vi "move_andor_files.vi"(8 "error in":errorcluster, 10 "Data Files Path":path, 11 "Andor setup":T1) -> (0 "error out":errorcluster)   [LabVIEW 2012]
uses:
  Andor_settings.ctl
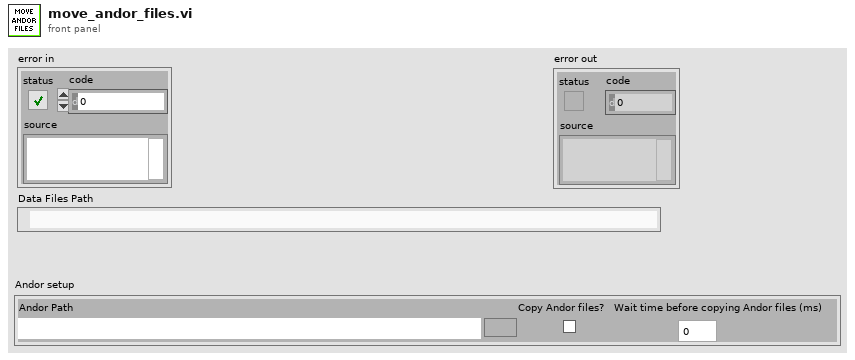
[diagram p1: front panel]
types:
  T1 = typedef "Andor_settings.ctl" = cluster{"Andor Path":path, "Copy any Andor files":bool, "Wait time before copying Andor files (ms)":u16}
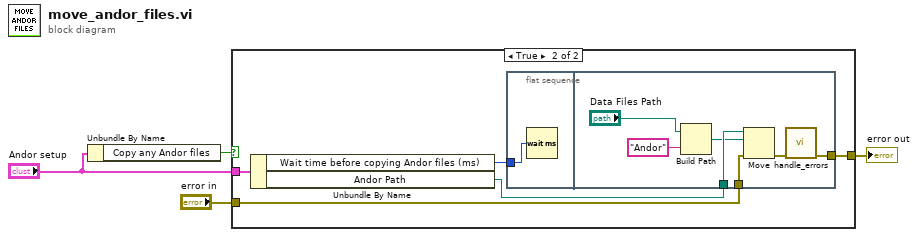
[diagram p0: block diagram]
diagram:
  n1 = Unbundle By Name("Andor setup") -> ("Copy any Andor files"=w4:bool)
  n2 = case shown="True" w4 {
    tunnel: "Andor setup" -> [_ w10]
    tunnel: "error in" -> [w5 w7]
    tunnel: [w5 w6] -> w1
    frame False {
    }
    frame True {
      n3 = Unbundle By Name(w10) -> ("Wait time before copying Andor files (ms)"=w9:u16, "Andor Path"=w8:path)
      n4 = flat-sequence {
        tunnel: w9 -> [w11]
        tunnel: w8 -> [w18]
        tunnel: w7 -> [w16]
        tunnel: [w15] -> w6
        frame #0 {
          n5 = Wait (ms)(milliseconds to wait=w11) -> ()  [unwired: 1 out]
        }
        frame #1 {
          n6 = Build Path(base path="Data Files Path", name or relative path="Andor") -> (appended path=w12:path)
          n7 = Move(source path=w18, error in=w16, 10:w12) -> (error out=w17:errorcluster)  [unwired: 2 in, 2 out]
          n8 = call "handle_errors.vi"("error in (no error)"=w17) -> ("error out"=w15:errorcluster)  [unwired: 9 in, 1 out]
        }
      }
    }
  }
  "error out" <- w1
